vi "PC Main.vi"() -> ()   [LabVIEW 2021]
uses:
  <vilib>/nisyscfg/Close (System).vi
  <vilib>/nisyscfg/nisyscfg.lvlib
panel:
  in  "Target IP":string
  out "current time":timestamp
  in  "Restart":bool
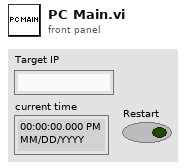
[diagram p1: front panel]
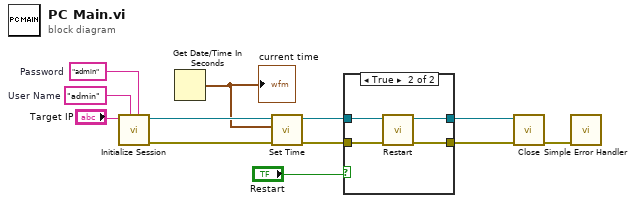
[diagram p0: block diagram]
diagram:
  w2 = "admin"  # Password
  w3 = "admin"  # User Name
  n1 = call <vilib>:"Initialize Session.vi"("Password"=w2, "User Name"=w3, "Target (localhost)"="Target IP") -> ("error out"=w11:errorcluster, "Session out"=w12:refnum<k21>)  [unwired: 7 in]
  n2 = Get Date/Time In Seconds() -> (seconds since 1Jan1904=w5:timestamp)
  "current time" <- w5
  n3 = call <vilib>:"Set Time.vi"("error in (no error)"=w11, "Time"=w5, "Session in (localhost)"=w12) -> ("error out"=w9:errorcluster, "Session out"=w10:refnum<k21>)  [unwired: 5 in, 2 out]
  n4 = case shown="True" "Restart" {
    tunnel: w10 -> [w14 w18]
    tunnel: w9 -> [w13 w17]
    tunnel: [w14 w16] -> w8
    tunnel: [w13 w15] -> w7
    frame False {
    }
    frame True {
      n5 = call <vilib>:"Restart.vi"("error in (no error)"=w17, "Session in"=w18) -> ("error out"=w15:errorcluster, "Session out"=w16:refnum<k21>)  [unwired: 7 in, 1 out]
    }
  }
  n6 = call-poly <vilib>:"Close.vi"("error in (no error)"=w7, "Session in"=w8) -> ("error out"=w4:errorcluster)  [unwired: 9 in]
  n7 = call <vilib>:"Simple Error Handler.vi"("error in (no error)"=w4) -> ()  [unwired: 4 in, 5 out]
